vi "Config Alarm.vi"(0 "VISA resource name":refnum<visa-resource-name>, 1 "Source (0: Kelvin)":u16(ring) items=["Kelvin", "Ohms", "Linear Data"], 2 "High Value (0.00000E+0)":dbl min=0.0 max=100000000.0 step=1e-06 format="%^.5e", 5 "Channel (1)":i32=1 min=0 max=16 step=1, 7 "Alarm On/Off (F: Off)":bool, 9 "Latch Enable (F: Enable)":bool, 11 "error in (no error)":errorcluster, 12 "Low Value (0.00000E+0)":dbl min=0.0 max=100000000.0 step=1e-06 format="%^.5e", 13 "Deadband (0.00000E+0)":dbl min=0.0 max=100000000.0 step=1e-06 format="%^.5e") -> (4 "VISA resource name out":refnum<visa-resource-name>, 15 "error out":errorcluster)   [LabVIEW 2012, in "Lake Shore Cryotronics 370.lvlib"]
doc: "This VI configures the 370 alarm functions. Control is provided over the alarm high and low setpoints, trigger inside/outside status, audible alarm status, and alarm active status. A display annunciator and audible beeper signal an active alarm at the instrument."
uses:
  <instrlib>/Lake Shore Cryotronics 370/Lake Shore Cryotronics 370.lvlib
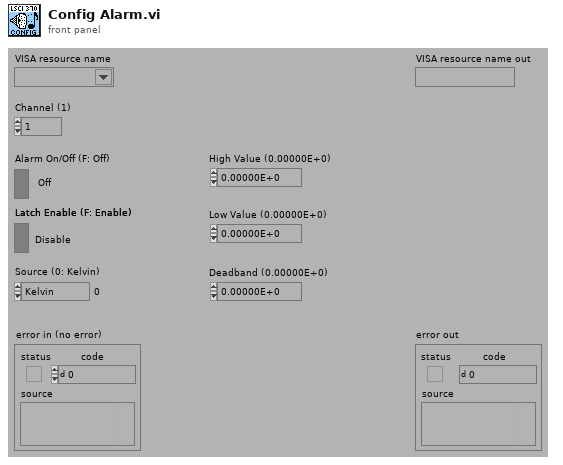
[diagram p1: front panel]
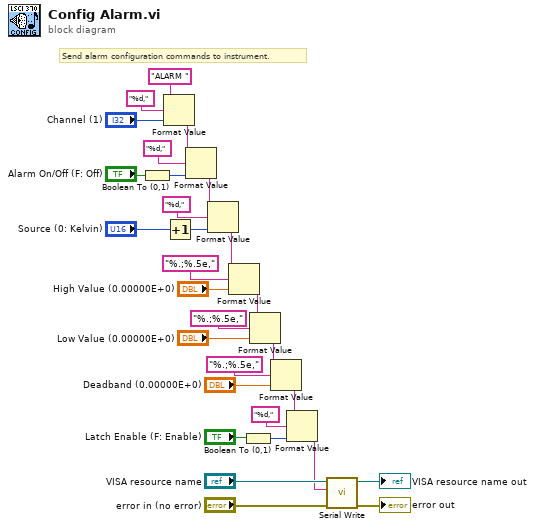
[diagram p0: block diagram]
diagram:
  # "Send alarm configuration commands to instrument."
  n1 = Boolean To (0,1)(Boolean="Alarm On/Off (F: Off)") -> (0, 1=w23:i16)
  n2 = Format Value(string ("")="ALARM ", format string="%d,", value (0)="Channel (1)") -> (output string=w5:string)
  n3 = Increment(x="Source (0: Kelvin)") -> (x+1=w20:u16)
  n4 = Format Value(string ("")=w5, format string="%d,", value (0)=w23) -> (output string=w19:string)
  n5 = Format Value(string ("")=w19, format string="%d,", value (0)=w20) -> (output string=w17:string)
  n6 = Format Value(string ("")=w17, format string="%.;%.5e,", value (0)="High Value (0.00000E+0)") -> (output string=w14:string)
  n7 = Boolean To (0,1)(Boolean="Latch Enable (F: Enable)") -> (0, 1=w13:i16)
  n8 = Format Value(string ("")=w14, format string="%.;%.5e,", value (0)="Low Value (0.00000E+0)") -> (output string=w9:string)
  n9 = Format Value(string ("")=w9, format string="%.;%.5e,", value (0)="Deadband (0.00000E+0)") -> (output string=w8:string)
  n10 = Format Value(string ("")=w8, format string="%d,", value (0)=w13) -> (output string=w7:string)
  n11 = call <instrlib>:"Serial Write.vi"("error in (no error)"="error in (no error)", "Write Buffer (\"\")"=w7, "VISA resource name"="VISA resource name") -> ("error out"=→"error out":errorcluster, "VISA resource name out"=→"VISA resource name out":refnum<visa-resource-name>)  [unwired: 6 in, 1 out]
